vi "insert_edge.vi"(10 "edge":refnum<class "Edge.lvclass">, 11 "digraph":refnum<class "Graph.lvclass">) -> (1 "edge unchanged?":bool, 2 "edge already included?":bool, 3 "digraph out":refnum<class "Graph.lvclass">)   [LabVIEW 2020, in "graph.lvlib" / "Graph.lvclass"]
uses:
  Graph.lvclass
  Edge/Edge.lvclass
  Graph.lvclass/Graph.ctl
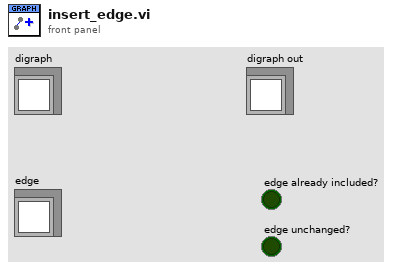
[diagram p1: front panel]
types:
  T1 = typedef "graph.lvlib/Graph.lvclass/edge-definition-cluster.ctl" = cluster{"source-id":refnum<class "ID.lvclass">, "sink-id":refnum<class "ID.lvclass">}
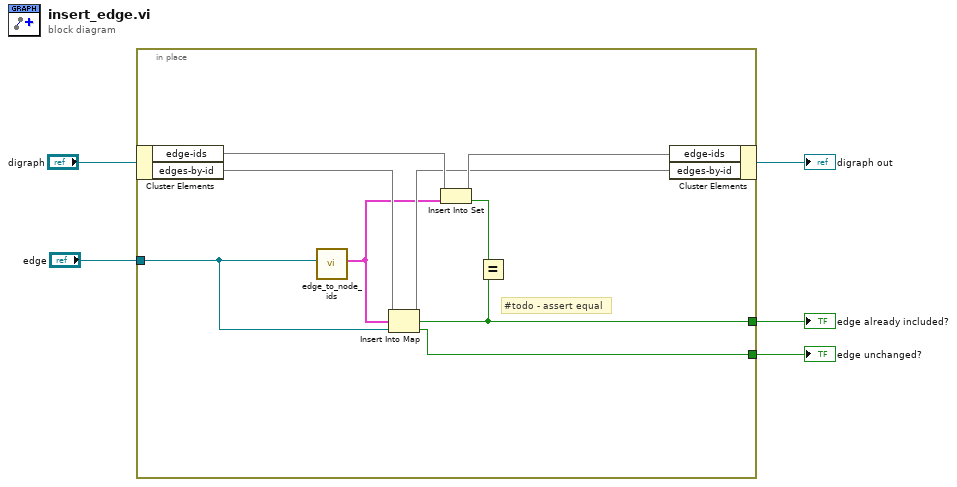
[diagram p0: block diagram]
diagram:
  n1 = in-place {
    in-place-border: [w6] -> w1
    in-place-border: "edge" -> [w9]
    in-place-border: [w7] -> w3
    # "#todo - assert equal"
    n2 = in-place-cluster #1("digraph") -> ("edge-ids"=w14:set{T1}, "edges-by-id"=w11:map{T1, refnum<class "Edge.lvclass">})
    n3 = call "edge_to_node_ids.vi"("edge"=w9) -> ("node-ids-cluster"=w10:T1)  [unwired: 10 in]
    n4 = Insert Into Map(map in=w11, key=w10, value=w9) -> (map out=w12:map{T1, refnum<class "Edge.lvclass">}, key already included?=w6:bool, value unchanged?=w7:bool)
    n5 = Insert Into Set(10:w10, 11:w14) -> (2:w8:bool, 3:w13:set{T1})
    n6 = Equal?(x=w8, y=w6) -> ()  [unwired: 1 out]
    n7 = in-place-cluster #1("edge-ids"=w13, "edges-by-id"=w12) -> (→"digraph out":refnum<class "Graph.lvclass">)
  }
  "edge unchanged?" <- w3
  "edge already included?" <- w1
